vi "GEA2 Flash APL.vi"(0 "GEA2 Reference In":refnum<k24>, 2 "Force Update?":bool, 5 "Source Address":u8=228 format="%.0x", 7 "Destination Address":u8 format="%.0x", 9 "File Path":path, 11 "Error In":errorcluster, 12 "Broadcast":bool=TRUE, 13 "Reset?":bool=TRUE) -> (4 "GEA2 Reference Out":refnum<k24>, 6 "Result":i32(ring) items=["ImageRejected", "BoardNotFound", "UnableToGetGeaConfiguration", "WriteToFlashNotAllowed", "ImageDownloadedSuccessfully", "ImagePresent", "WriteToFlashFailed", "EraseFailed", "CrcFailed"], 8 "Pass/Fail":bool, 10 "Report Text":string, 15 "Error Out":errorcluster)   [LabVIEW 2020, in "GEA2_Toolkit.lvlib"]
doc: "This VI will flash an APL file onto an appliance board. The input 'Filename' accepts a string with file extension, for example 'MC_v1.06.apl'. Force Update will ensure the APL is downloaded even if it is the same version as what already exists on the appliance board."
uses:
  library/GEA2_Toolkit.lvlib
  C:/TechnologyLab/NI-2010/Drivers/GEA3 Toolkit/GEA3 DLL Source/GeaCommunication.dll
  GEA3 DLL Source/GeaCommunication.dll
  C:/TechnologyLab/NI-2010/Drivers/GEA3 Toolkit/GEA3 DLL Source/Programming.dll
  GEA3 DLL Source/Programming.dll
  C:/TechnologyLab/NI-2010/Drivers/GEA3 Toolkit/GEA3 DLL Source/Encoding.dll
  GEA3 DLL Source/Encoding.dll
panel:
  in  "Time to Enter BL (ms)":u16=5000
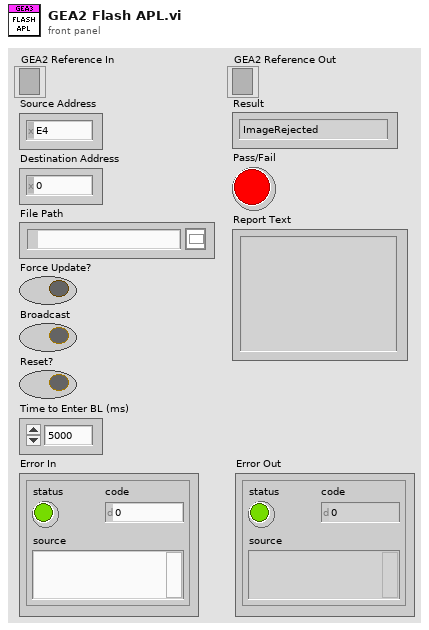
[diagram p1: front panel]
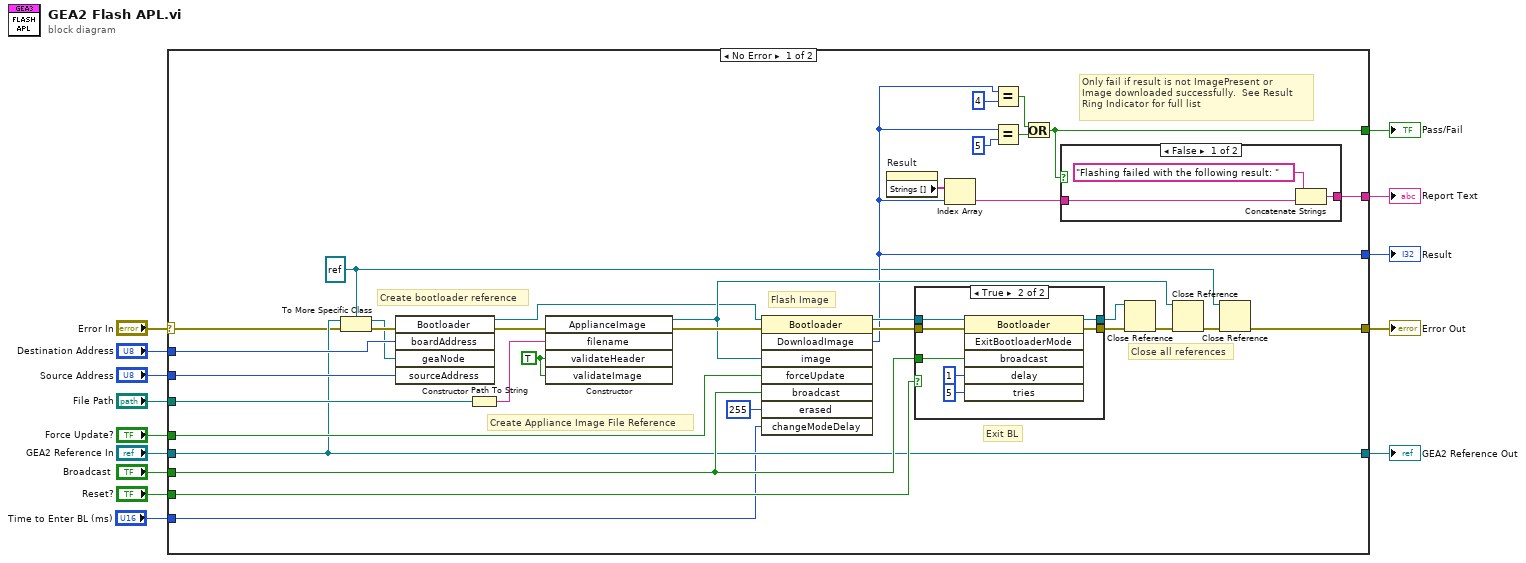
[diagram p0: block diagram]
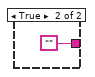
[diagram p3: hidden frame]
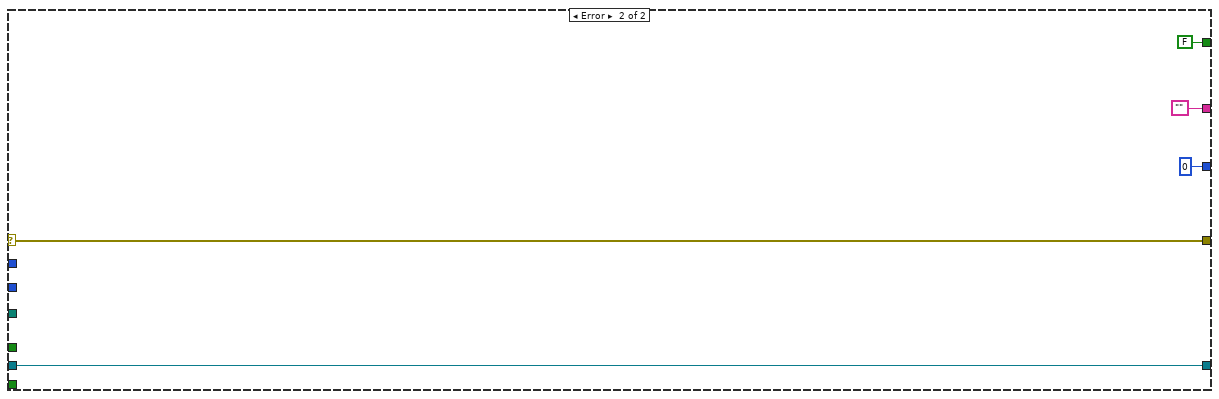
[diagram p4: hidden frame]
diagram:
  n1 = case shown="No Error" "Error In" {
    selector: "Error In" -> [w26 w66]
    tunnel: "GEA2 Reference In" -> [w27 w67]
    tunnel: "Destination Address" -> [w49 _]
    tunnel: "Force Update?" -> [w30 _]
    tunnel: "Source Address" -> [w32 _]
    tunnel: [w23 0 ("DownloadImage")] -> w2
    tunnel: [w19 w66] -> w10
    tunnel: [w27 w67] -> w9
    tunnel: "File Path" -> [w41 _]
    tunnel: "Broadcast" -> [w29 _]
    tunnel: [w36 FALSE] -> w6
    tunnel: [w34 ""] -> w5
    tunnel: "Reset?" -> [w33 _]
    tunnel: "Time to Enter BL (ms)" -> [w18 _]
    frame No Error {
      w16 = TRUE ("validateHeader")
      w20 = refnum<k24> refnum ("geaNode")
      # "Only fail if result is not ImagePresent or\nImage downloaded successfully.  See Result\nRing Indicator for full list"
      # "Exit BL"
      # "Flash Image"
      # "Create Appliance Image File Reference"
      # "Close all references"
      # "Create bootloader reference"
      n2 = To More Specific Class(target class=w20, reference=w27, error in=w26) -> (specific class reference=w24:refnum<k24>, error out=w25:errorcluster)
      n3 = constructor class="Bootloader"(error in=w25, "boardAddress"=w49, "geaNode"=w24, "sourceAddress"=w32) -> (reference out=w15:refnum<k24>, error out=w17:errorcluster)  [unwired: 2 in, 4 out]
      n4 = Path To String(path=w41) -> (string=w42:string)
      n5 = constructor class="ApplianceImage"(error in=w17, "filename"=w42, "validateHeader"=w16, "validateImage"=w16) -> (reference out=w28:refnum<k24>, error out=w48:errorcluster)  [unwired: 2 in, 4 out]
      n6 = invoke class="Bootloader" method="DownloadImage"(reference=w15, error in=w48, "image"=w28, "forceUpdate"=w30, "broadcast"=w29, "erased"=u8 255, "changeModeDelay"=w18) -> (reference out=w46:refnum<k24>, error out=w45:errorcluster, "DownloadImage"=w23:i32)  [unwired: 1 in, 5 out]
      n7 = property on="Result" class="Ring (strict)"() -> ("Strings []"=w22:string[])  [unwired: 2 in, 2 out]
      n8 = case shown="True" w33 {
        tunnel: w46 -> [w50 w58]
        tunnel: w45 -> [w51 w57]
        tunnel: [w50 w56] -> w44
        tunnel: [w51 w55] -> w43
        tunnel: w29 -> [_ w54]
        frame False {
        }
        frame True {
          n9 = invoke class="Bootloader" method="ExitBootloaderMode"(reference=w58, error in=w57, "broadcast"=w54, "delay"=u8 1, "tries"=u8 5) -> (reference out=w56:refnum<k24>, error out=w55:errorcluster)  [unwired: 1 in, 4 out]
        }
      }
      n10 = Index Array(array=w22, index=w23) -> (element=w35:string)
      n11 = Equal?(x=w23, y=4) -> (x = y?=w39:bool)
      n12 = Equal?(x=w23, y=5) -> (x = y?=w40:bool)
      n13 = Or(x=w39, y=w40) -> (x .or. y?=w36:bool)
      n14 = case shown="False" w36 {
        tunnel: w35 -> [w60 _]
        tunnel: [w59 ""] -> w34
        frame False {
          n15 = Concatenate Strings("Flashing failed with the following result: ", w60) -> (w59:string)
        }
        frame True {
        }
      }
      n16 = Close Reference(reference=w44, error in (no error)=w43) -> (error out=w47:errorcluster)
      n17 = Close Reference(reference=w28, error in (no error)=w47) -> (error out=w21:errorcluster)
      n18 = Close Reference(reference=w20, error in (no error)=w21) -> (error out=w19:errorcluster)
    }
    frame Error {
    }
  }
  "GEA2 Reference Out" <- w9
  "Error Out" <- w10
  "Pass/Fail" <- w6
  "Report Text" <- w5
  "Result" <- w2
